vi "test-swerve-drve-odometry-01.vi"() -> (3 "Test Passed":bool)   [LabVIEW 2019]
uses:
  <vilib>/Rock Robotics/WPI/ThirdParty/JAS_Junk/TrajLib/TypeDef/SWERVE_DRIVE_ODOMETRY.ctl
  <vilib>/Rock Robotics/WPI/ThirdParty/JAS_Junk/TrajLib/TypeDef/POSE2D.ctl
  <vilib>/Rock Robotics/WPI/ThirdParty/JAS_Junk/TrajLib/TypeDef/TRANSLATION2D.ctl
  <vilib>/Rock Robotics/WPI/ThirdParty/JAS_Junk/TrajLib/TypeDef/ROTATION2D.ctl
  <vilib>/Rock Robotics/WPI/ThirdParty/JAS_Junk/TrajLib/TypeDef/SWERVE_DRIVE_MODULE_POSITION.ctl
  <vilib>/Rock Robotics/WPI/ThirdParty/JAS_Junk/TrajLib/TypeDef/SWERVE_DRIVE_KINEMATICS.ctl
  <vilib>/Analysis/Matrix/Datatypes/RealMatrix.ctl
  <vilib>/Rock Robotics/WPI/ThirdParty/JAS_Junk/TrajLib/TypeDef/SWERVE_DRIVE_MODULE_STATE.ctl
  <vilib>/Rock Robotics/WPI/ThirdParty/JAS_Junk/TrajLib/Conv_Deg_Radians.vi
  <vilib>/Rock Robotics/WPI/ThirdParty/JAS_Junk/TrajLib/Rotation2d_CreateAngle.vi
  <vilib>/Rock Robotics/WPI/ThirdParty/JAS_Junk/TrajLib/Trajectory_Library.lvlib
  <vilib>/Analysis/Matrix/NI_Matrix.lvlib
panel:
  out "Odom 1":T1={"POSE"={"TRANSLATION"={"X"=0.0, "Y"=0.0}, "ROTATION"={"VALUE"=0.0, "COS"=1.0, "SIN"=0.0}}, "GyroOffset"={"VALUE"=0.0, "COS"=1.0, "SIN"=0.0}, "PreviousAngle"={"VALUE"=0.0, "COS"=1.0, "SIN"=0.0}, "PrevModulePositions"=[], "NumModules"=0} {"PrevModulePositions"."Angle"."SIN" format="%13.4f"; "PrevModulePositions"."Angle"."COS" format="%13.4f"; "PrevModulePositions"."Angle"."VALUE" format="%13.4f"; "PreviousAngle"."SIN" format="%13.4f"; "PreviousAngle"."COS" format="%13.4f"; "PreviousAngle"."VALUE" format="%13.4f"; "GyroOffset"."SIN" format="%13.4f"; "GyroOffset"."COS" format="%13.4f"; "GyroOffset"."VALUE" format="%13.4f"; "POSE"."ROTATION"."SIN" format="%13.4f"; "POSE"."ROTATION"."COS" format="%13.4f"; "POSE"."ROTATION"."VALUE" format="%13.4f"; "POSE"."TRANSLATION"."Y" format="%14.3f"; "POSE"."TRANSLATION"."X" format="%14.3f"}
  out "robot POSE 4":T2={"TRANSLATION"={"X"=0.0, "Y"=0.0}, "ROTATION"={"VALUE"=0.0, "COS"=1.0, "SIN"=0.0}} {"ROTATION"."SIN" format="%13.4f"; "ROTATION"."COS" format="%13.4f"; "ROTATION"."VALUE" format="%13.4f"; "TRANSLATION"."Y" format="%14.3f"; "TRANSLATION"."X" format="%14.3f"}
  out "Odom 4":T1={"POSE"={"TRANSLATION"={"X"=0.0, "Y"=0.0}, "ROTATION"={"VALUE"=0.0, "COS"=1.0, "SIN"=0.0}}, "GyroOffset"={"VALUE"=0.0, "COS"=1.0, "SIN"=0.0}, "PreviousAngle"={"VALUE"=0.0, "COS"=1.0, "SIN"=0.0}, "PrevModulePositions"=[], "NumModules"=0} {"PrevModulePositions"."Angle"."SIN" format="%13.4f"; "PrevModulePositions"."Angle"."COS" format="%13.4f"; "PrevModulePositions"."Angle"."VALUE" format="%13.4f"; "PreviousAngle"."SIN" format="%13.4f"; "PreviousAngle"."COS" format="%13.4f"; "PreviousAngle"."VALUE" format="%13.4f"; "GyroOffset"."SIN" format="%13.4f"; "GyroOffset"."COS" format="%13.4f"; "GyroOffset"."VALUE" format="%13.4f"; "POSE"."ROTATION"."SIN" format="%13.4f"; "POSE"."ROTATION"."COS" format="%13.4f"; "POSE"."ROTATION"."VALUE" format="%13.4f"; "POSE"."TRANSLATION"."Y" format="%14.3f"; "POSE"."TRANSLATION"."X" format="%14.3f"}
  out "SWERVE_DRIVE_KINEMATICS":T6 {"SavedModuleStates"."Angle"."SIN" format="%13.4f"; "SavedModuleStates"."Angle"."COS" format="%13.4f"; "SavedModuleStates"."Angle"."VALUE" format="%13.4f"; "PrevCoR"."Y" format="%14.3f"; "PrevCoR"."X" format="%14.3f"; "Modules"."Y" format="%14.3f"; "Modules"."X" format="%14.3f"}
  out "robot POSE 3":T2={"TRANSLATION"={"X"=0.0, "Y"=0.0}, "ROTATION"={"VALUE"=0.0, "COS"=1.0, "SIN"=0.0}} {"ROTATION"."SIN" format="%13.4f"; "ROTATION"."COS" format="%13.4f"; "ROTATION"."VALUE" format="%13.4f"; "TRANSLATION"."Y" format="%14.3f"; "TRANSLATION"."X" format="%14.3f"}
  out "Odom 3":T1={"POSE"={"TRANSLATION"={"X"=0.0, "Y"=0.0}, "ROTATION"={"VALUE"=0.0, "COS"=1.0, "SIN"=0.0}}, "GyroOffset"={"VALUE"=0.0, "COS"=1.0, "SIN"=0.0}, "PreviousAngle"={"VALUE"=0.0, "COS"=1.0, "SIN"=0.0}, "PrevModulePositions"=[], "NumModules"=0} {"PrevModulePositions"."Angle"."SIN" format="%13.4f"; "PrevModulePositions"."Angle"."COS" format="%13.4f"; "PrevModulePositions"."Angle"."VALUE" format="%13.4f"; "PreviousAngle"."SIN" format="%13.4f"; "PreviousAngle"."COS" format="%13.4f"; "PreviousAngle"."VALUE" format="%13.4f"; "GyroOffset"."SIN" format="%13.4f"; "GyroOffset"."COS" format="%13.4f"; "GyroOffset"."VALUE" format="%13.4f"; "POSE"."ROTATION"."SIN" format="%13.4f"; "POSE"."ROTATION"."COS" format="%13.4f"; "POSE"."ROTATION"."VALUE" format="%13.4f"; "POSE"."TRANSLATION"."Y" format="%14.3f"; "POSE"."TRANSLATION"."X" format="%14.3f"}
  out "Odom 0":T1={"POSE"={"TRANSLATION"={"X"=0.0, "Y"=0.0}, "ROTATION"={"VALUE"=0.0, "COS"=1.0, "SIN"=0.0}}, "GyroOffset"={"VALUE"=0.0, "COS"=1.0, "SIN"=0.0}, "PreviousAngle"={"VALUE"=0.0, "COS"=1.0, "SIN"=0.0}, "PrevModulePositions"=[], "NumModules"=0} {"PrevModulePositions"."Angle"."SIN" format="%13.4f"; "PrevModulePositions"."Angle"."COS" format="%13.4f"; "PrevModulePositions"."Angle"."VALUE" format="%13.4f"; "PreviousAngle"."SIN" format="%13.4f"; "PreviousAngle"."COS" format="%13.4f"; "PreviousAngle"."VALUE" format="%13.4f"; "GyroOffset"."SIN" format="%13.4f"; "GyroOffset"."COS" format="%13.4f"; "GyroOffset"."VALUE" format="%13.4f"; "POSE"."ROTATION"."SIN" format="%13.4f"; "POSE"."ROTATION"."COS" format="%13.4f"; "POSE"."ROTATION"."VALUE" format="%13.4f"; "POSE"."TRANSLATION"."Y" format="%14.3f"; "POSE"."TRANSLATION"."X" format="%14.3f"}
  out "robot POSE 0":T2={"TRANSLATION"={"X"=0.0, "Y"=0.0}, "ROTATION"={"VALUE"=0.0, "COS"=1.0, "SIN"=0.0}} {"ROTATION"."SIN" format="%13.4f"; "ROTATION"."COS" format="%13.4f"; "ROTATION"."VALUE" format="%13.4f"; "TRANSLATION"."Y" format="%14.3f"; "TRANSLATION"."X" format="%14.3f"}
  out "robot POSE 1":T2={"TRANSLATION"={"X"=0.0, "Y"=0.0}, "ROTATION"={"VALUE"=0.0, "COS"=1.0, "SIN"=0.0}} {"ROTATION"."SIN" format="%13.4f"; "ROTATION"."COS" format="%13.4f"; "ROTATION"."VALUE" format="%13.4f"; "TRANSLATION"."Y" format="%14.3f"; "TRANSLATION"."X" format="%14.3f"}
  out "robot POSE 2":T2={"TRANSLATION"={"X"=0.0, "Y"=0.0}, "ROTATION"={"VALUE"=0.0, "COS"=1.0, "SIN"=0.0}} {"ROTATION"."SIN" format="%13.4f"; "ROTATION"."COS" format="%13.4f"; "ROTATION"."VALUE" format="%13.4f"; "TRANSLATION"."Y" format="%14.3f"; "TRANSLATION"."X" format="%14.3f"}
  out "Odom 2":T1={"POSE"={"TRANSLATION"={"X"=0.0, "Y"=0.0}, "ROTATION"={"VALUE"=0.0, "COS"=1.0, "SIN"=0.0}}, "GyroOffset"={"VALUE"=0.0, "COS"=1.0, "SIN"=0.0}, "PreviousAngle"={"VALUE"=0.0, "COS"=1.0, "SIN"=0.0}, "PrevModulePositions"=[], "NumModules"=0} {"PrevModulePositions"."Angle"."SIN" format="%13.4f"; "PrevModulePositions"."Angle"."COS" format="%13.4f"; "PrevModulePositions"."Angle"."VALUE" format="%13.4f"; "PreviousAngle"."SIN" format="%13.4f"; "PreviousAngle"."COS" format="%13.4f"; "PreviousAngle"."VALUE" format="%13.4f"; "GyroOffset"."SIN" format="%13.4f"; "GyroOffset"."COS" format="%13.4f"; "GyroOffset"."VALUE" format="%13.4f"; "POSE"."ROTATION"."SIN" format="%13.4f"; "POSE"."ROTATION"."COS" format="%13.4f"; "POSE"."ROTATION"."VALUE" format="%13.4f"; "POSE"."TRANSLATION"."Y" format="%14.3f"; "POSE"."TRANSLATION"."X" format="%14.3f"}
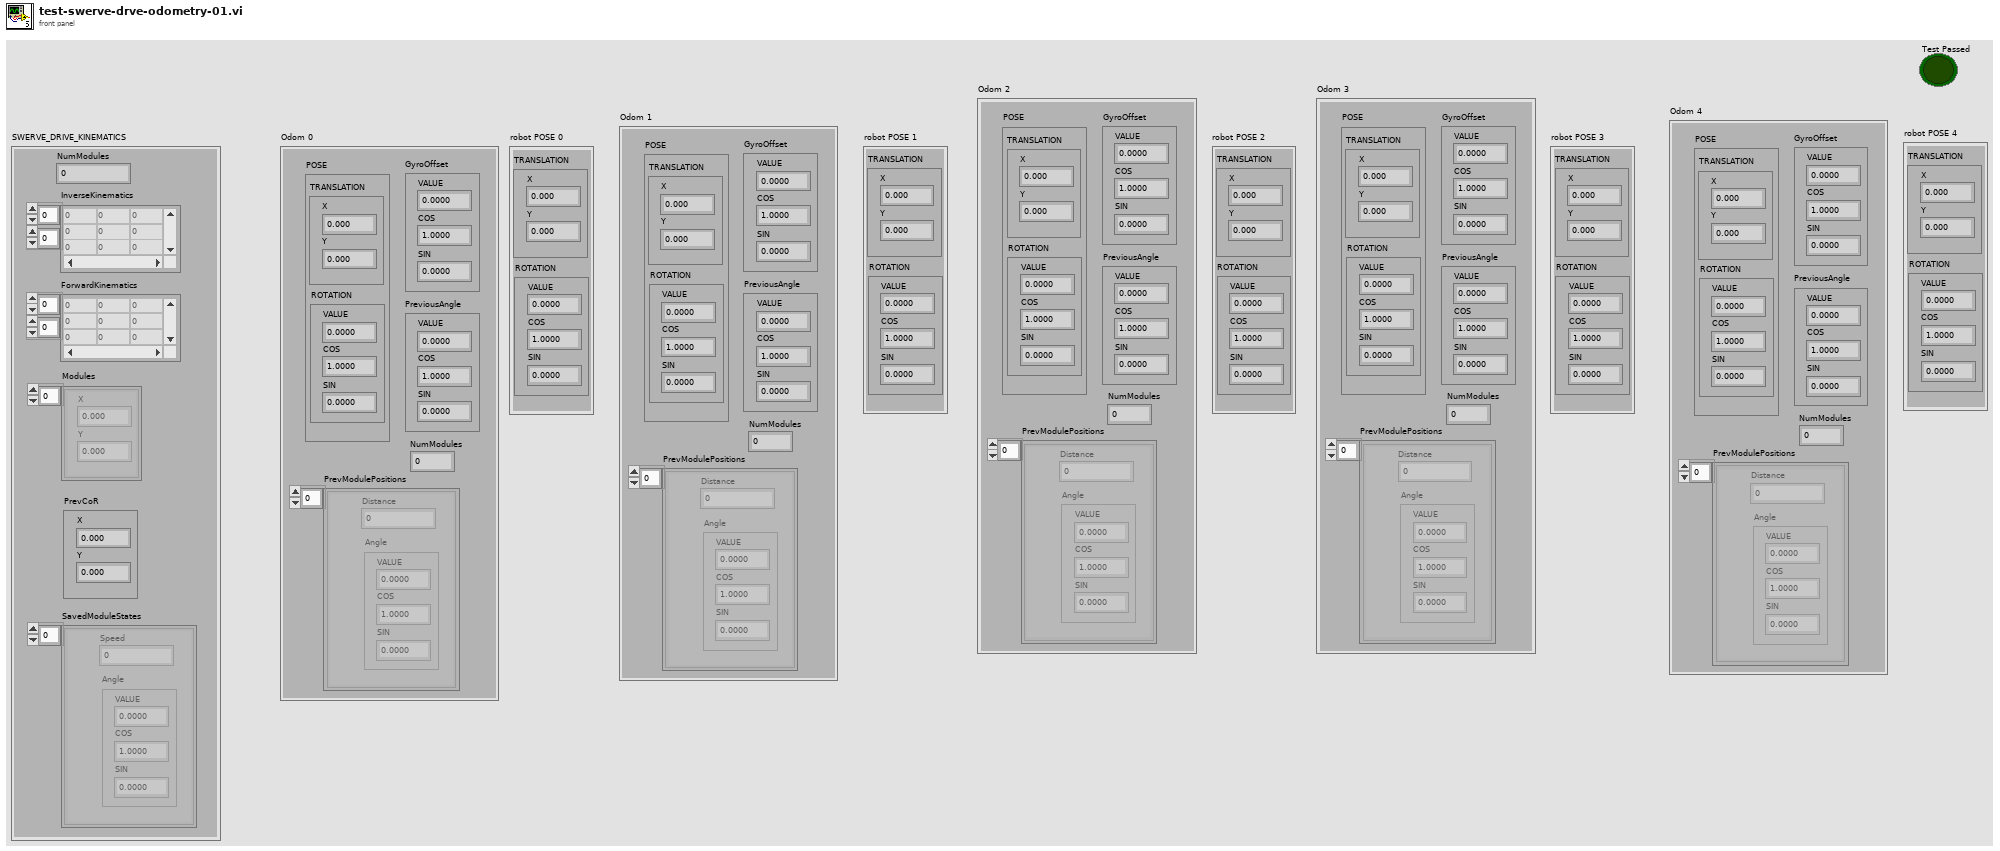
[diagram p1: front panel]
types:
  T1 = typedef "Trajectory_Library.lvlib/SWERVE_DRIVE_ODOMETRY.ctl" = cluster{"POSE":T2, "GyroOffset":T4, "PreviousAngle":T4, "PrevModulePositions":T5[], "NumModules":i32}
  T2 = typedef "Trajectory_Library.lvlib/POSE2D.ctl" = cluster{"TRANSLATION":T3, "ROTATION":T4}
  T3 = typedef "Trajectory_Library.lvlib/TRANSLATION2D.ctl" = cluster{"X":dbl, "Y":dbl}
  T4 = typedef "Trajectory_Library.lvlib/ROTATION2D.ctl" = cluster{"VALUE":dbl, "COS":dbl, "SIN":dbl}
  T5 = typedef "Trajectory_Library.lvlib/SWERVE_DRIVE_MODULE_POSITION.ctl" = cluster{"Distance":dbl, "Angle":T4}
  T6 = typedef "Trajectory_Library.lvlib/SWERVE_DRIVE_KINEMATICS.ctl" = cluster{"NumModules":i32, "InverseKinematics":T7, "ForwardKinematics":T7, "Modules":T3[], "PrevCoR":T3, "SavedModuleStates":T8[]}
  T7 = typedef "NI_Matrix.lvlib/RealMatrix.ctl" = dbl[][]
  T8 = typedef "Trajectory_Library.lvlib/SWERVE_DRIVE_MODULE_STATE.ctl" = cluster{"Speed":dbl, "Angle":T4}
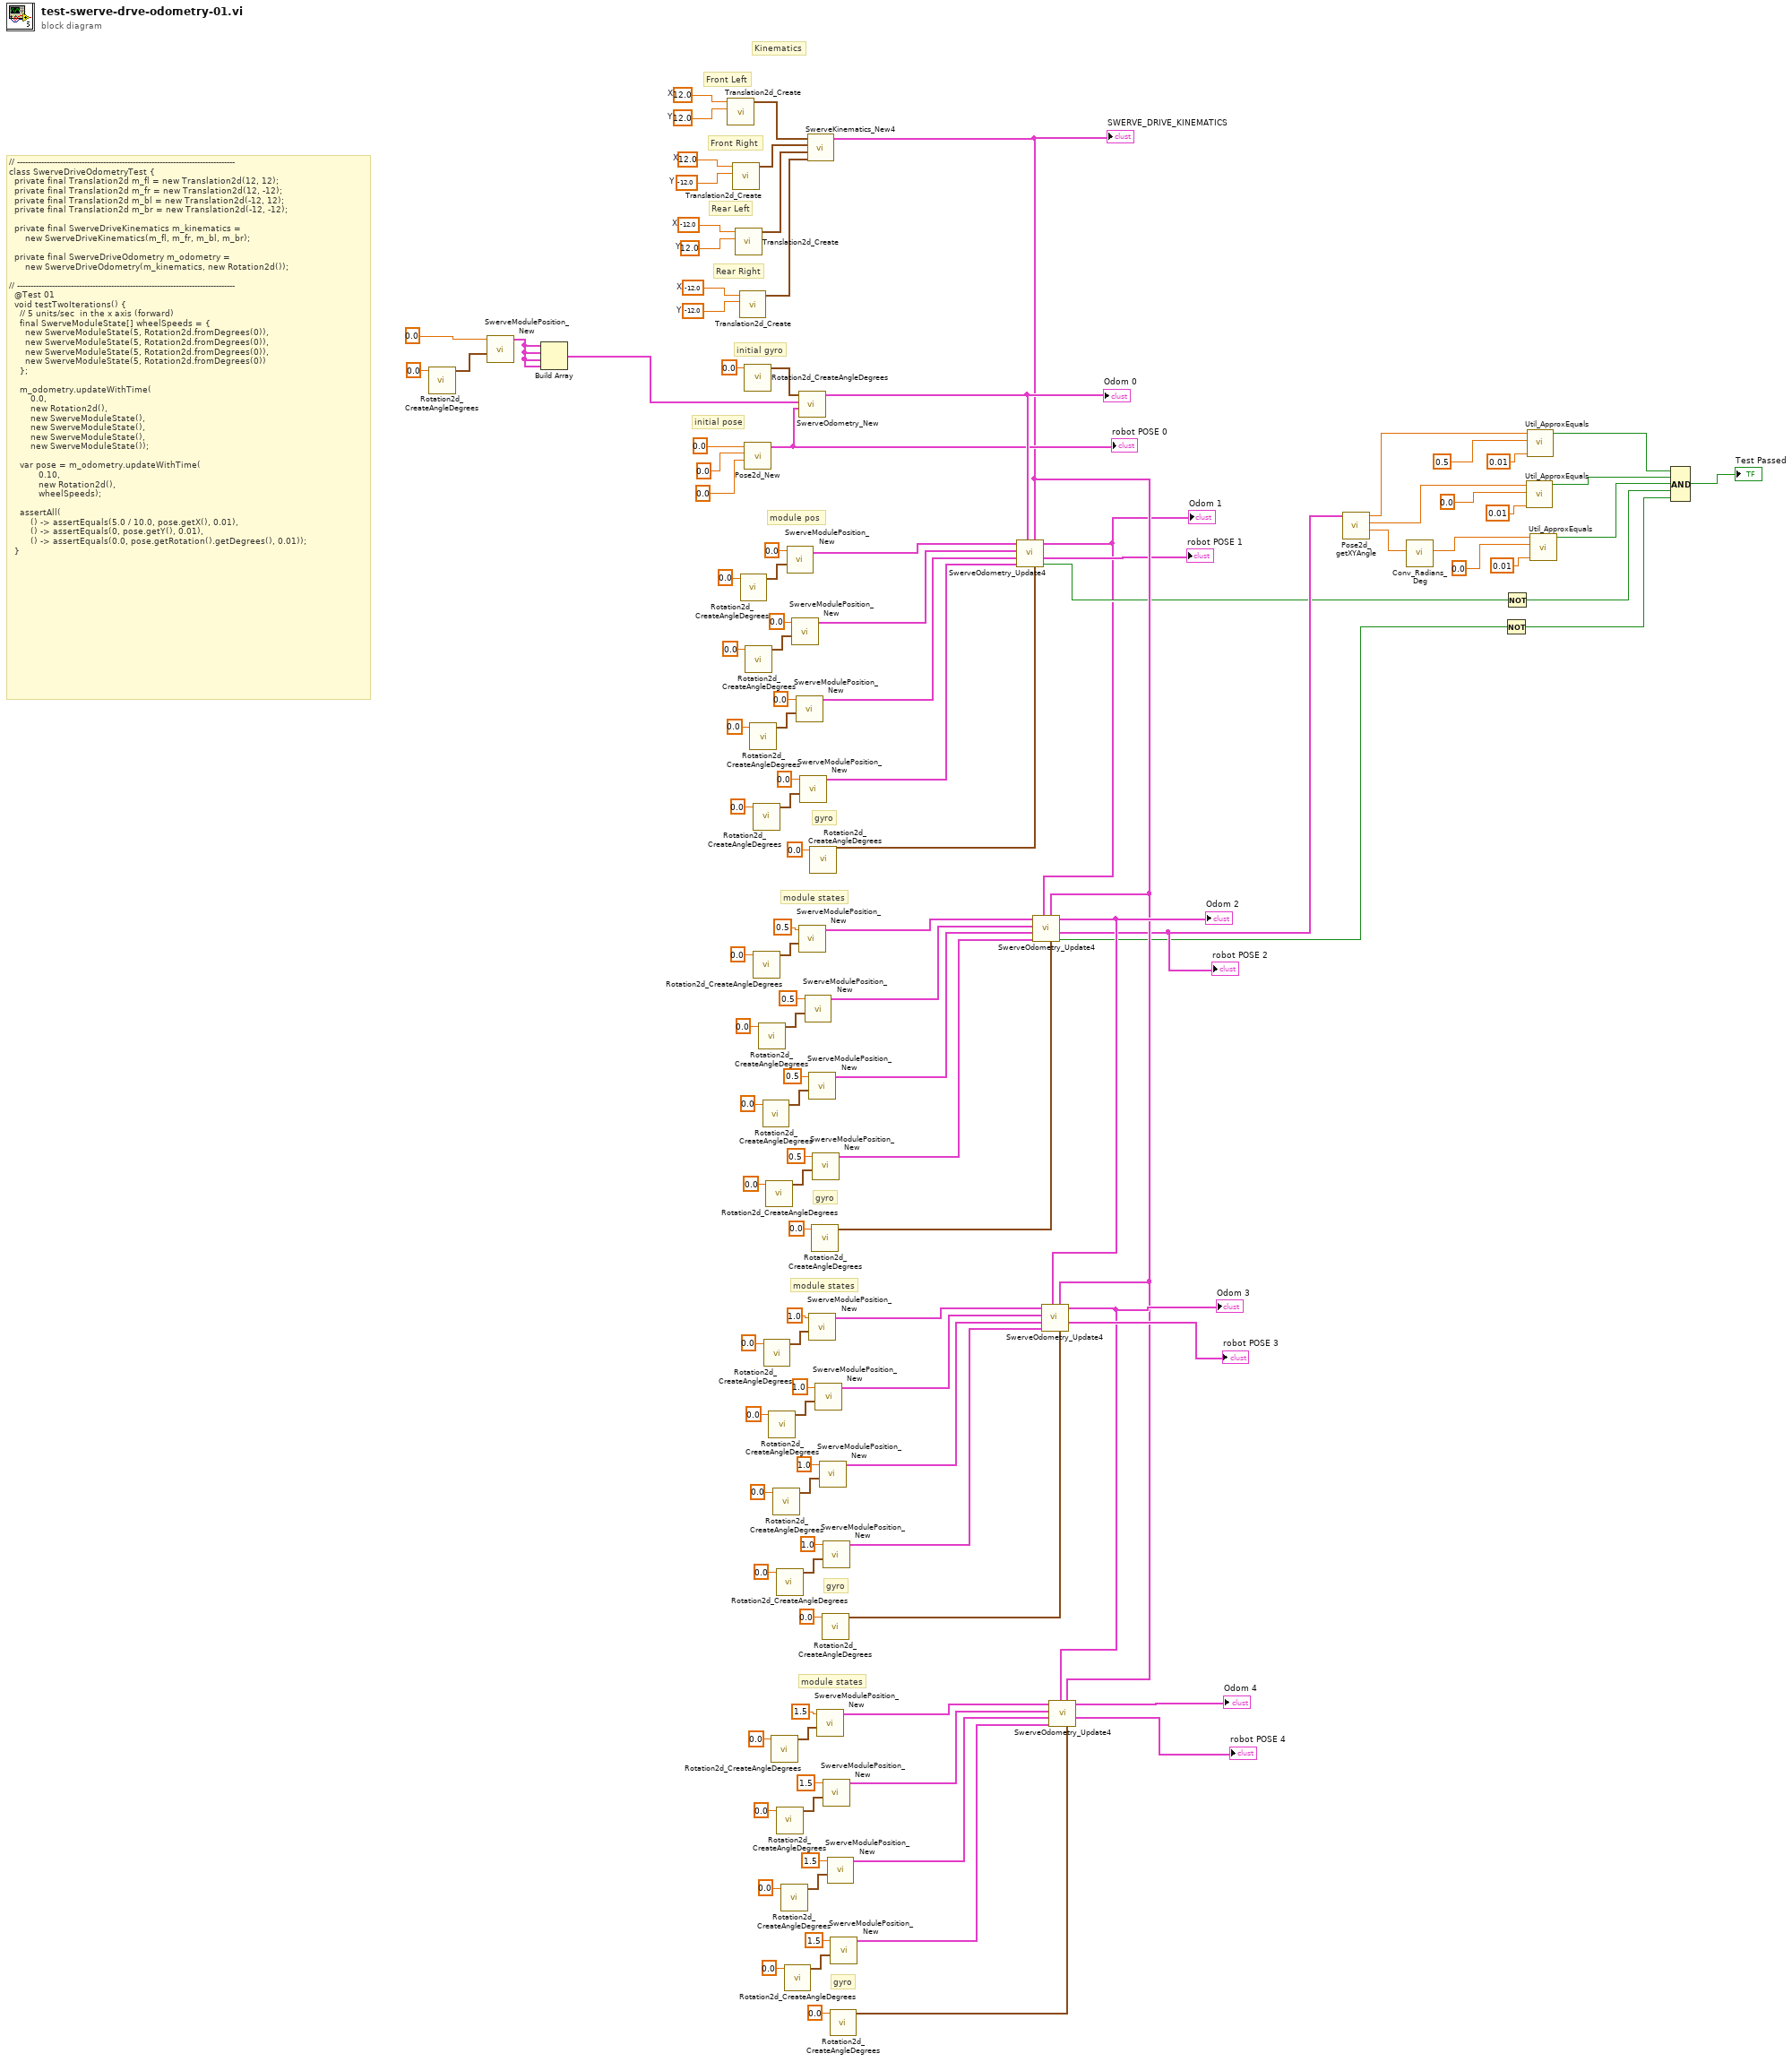
[diagram p0: block diagram]
diagram:
  w119 = -12.0  # X
  w118 = -12.0  # Y
  w117 = -12.0  # X
  w116 = 12.0  # Y
  w115 = 12.0  # X
  w114 = -12.0  # Y
  w113 = 12.0  # X
  w112 = 12.0  # Y
  # "gyro"
  # "module states"
  # "gyro"
  # "module states"
  # "initial pose"
  # "gyro"
  # "module states"
  # "gyro"
  # "module pos"
  # "Kinematics"
  # "initial gyro"
  # "Rear Right"
  # "Rear Left"
  # "Front Right"
  # "Front Left"
  # "// ---------------------------------------------------------------------------------\nclass SwerveDriveOdometryTest {\n  private final Translation2d m_fl = new Translation2d(12, 12);\n  private final Translation2d m_fr = new Translation2d(12, -12);\n  private final Translation2d m_bl = new Translation2d(-12, 12);\n  private final Translation2d m_br = new Translation2d(-12, -12);\n\n  private final SwerveDriveKinematics m_kinematics =\n      new SwerveDriveKinematics(m_fl, m_fr, m_bl, m_br);\n\n  private final SwerveDriveOdometry m_odometry =\n      new SwerveDriveOdometry(m_kinematics, new Rotation2d());\n\n// ---------------------------------------------------------------------------------\n  @Test 01\n  void testTwoIterations() {\n    // 5 units/sec  in the x axis (forward)\n    final SwerveModuleState[] wheelSpeeds = {\n      new SwerveModuleState(5, Rotation2d.fromDegrees(0)),\n      new SwerveModuleState(5, Rotation2d.fromDegrees(0)),\n      new SwerveModuleState(5, Rotation2d.fromDegrees(0)),\n      new SwerveModuleState(5, Rotation2d.fromDegrees(0))\n    };\n\n    m_odometry.updateWithTime(\n        0.0,\n        new Rotation2d(),\n        new SwerveModuleState(),\n        new SwerveModuleState(),\n        new SwerveModuleState(),\n        new SwerveModuleState());\n\n    var pose = m_odometry.updateWithTime(\n           0.10, \n           new Rotation2d(), \n           wheelSpeeds);\n\n    assertAll(\n        () -> assertEquals(5.0 / 10.0, pose.getX(), 0.01),\n        () -> assertEquals(0, pose.getY(), 0.01),\n        () -> assertEquals(0.0, pose.getRotation().getDegrees(), 0.01));\n  }"
  n1 = call <vilib>:"Rotation2d_CreateAngleDegrees.vi"("Angle_Degrees"=0.0) -> ("ROTATION"=w9:T4)  [unwired: 10 in]
  n2 = call <vilib>:"SwerveModulePosition_New.vi"("ROTATION"=w9, "Distance"=0.0) -> ("SWERVE_DRIVE_MODULE_POSITION"=w7:T5)  [unwired: 9 in]
  n3 = Build Array(w7, w7, w7, w7) -> (w6:T5[])
  n4 = call <vilib>:"Translation2d_Create.vi"("Y"=w112, "X"=w113) -> ("TRANSLATION"=w120:T3)  [unwired: 9 in]
  n5 = call <vilib>:"Translation2d_Create.vi"("Y"=w114, "X"=w115) -> ("TRANSLATION"=w121:T3)  [unwired: 9 in]
  n6 = call <vilib>:"Translation2d_Create.vi"("Y"=w116, "X"=w117) -> ("TRANSLATION"=w122:T3)  [unwired: 9 in]
  n7 = call <vilib>:"Translation2d_Create.vi"("Y"=w118, "X"=w119) -> ("TRANSLATION"=w123:T3)  [unwired: 9 in]
  n8 = call <vilib>:"Rotation2d_CreateAngleDegrees.vi"("Angle_Degrees"=0.0) -> ("ROTATION"=w105:T4)  [unwired: 10 in]
  n9 = call <vilib>:"Rotation2d_CreateAngleDegrees.vi"("Angle_Degrees"=0.0) -> ("ROTATION"=w108:T4)  [unwired: 10 in]
  n10 = call <vilib>:"Pose2d_New.vi"("Heading"=0.0, "Y"=0.0, "X"=0.0) -> ("out POSe"=w69:T2)  [unwired: 8 in]
  "robot POSE 0" <- w69
  n11 = call <vilib>:"Rotation2d_CreateAngleDegrees.vi"("Angle_Degrees"=0.0) -> ("ROTATION"=w102:T4)  [unwired: 10 in]
  n12 = call <vilib>:"Rotation2d_CreateAngleDegrees.vi"("Angle_Degrees"=0.0) -> ("ROTATION"=w99:T4)  [unwired: 10 in]
  n13 = call <vilib>:"Rotation2d_CreateAngleDegrees.vi"("Angle_Degrees"=0.0) -> ("ROTATION"=w96:T4)  [unwired: 10 in]
  n14 = call <vilib>:"Rotation2d_CreateAngleDegrees.vi"("Angle_Degrees"=0.0) -> ("ROTATION"=w89:T4)  [unwired: 10 in]
  n15 = call <vilib>:"Rotation2d_CreateAngleDegrees.vi"("Angle_Degrees"=0.0) -> ("ROTATION"=w86:T4)  [unwired: 10 in]
  n16 = call <vilib>:"Rotation2d_CreateAngleDegrees.vi"("Angle_Degrees"=0.0) -> ("ROTATION"=w83:T4)  [unwired: 10 in]
  n17 = call <vilib>:"Rotation2d_CreateAngleDegrees.vi"("Angle_Degrees"=0.0) -> ("ROTATION"=w67:T4)  [unwired: 10 in]
  n18 = call <vilib>:"Rotation2d_CreateAngleDegrees.vi"("Angle_Degrees"=0.0) -> ("ROTATION"=w80:T4)  [unwired: 10 in]
  n19 = call <vilib>:"Rotation2d_CreateAngleDegrees.vi"("Angle_Degrees"=0.0) -> ("ROTATION"=w64:T4)  [unwired: 10 in]
  n20 = call <vilib>:"Rotation2d_CreateAngleDegrees.vi"("Angle_Degrees"=0.0) -> ("ROTATION"=w47:T4)  [unwired: 10 in]
  n21 = call <vilib>:"Rotation2d_CreateAngleDegrees.vi"("Angle_Degrees"=0.0) -> ("ROTATION"=w61:T4)  [unwired: 10 in]
  n22 = call <vilib>:"Rotation2d_CreateAngleDegrees.vi"("Angle_Degrees"=0.0) -> ("ROTATION"=w58:T4)  [unwired: 10 in]
  n23 = call <vilib>:"Rotation2d_CreateAngleDegrees.vi"("Angle_Degrees"=0.0) -> ("ROTATION"=w44:T4)  [unwired: 10 in]
  n24 = call <vilib>:"Rotation2d_CreateAngleDegrees.vi"("Angle_Degrees"=0.0) -> ("ROTATION"=w41:T4)  [unwired: 10 in]
  n25 = call <vilib>:"Rotation2d_CreateAngleDegrees.vi"("Angle_Degrees"=0.0) -> ("ROTATION"=w38:T4)  [unwired: 10 in]
  n26 = call <vilib>:"SwerveModulePosition_New.vi"("ROTATION"=w105, "Distance"=0.0 ("Speed")) -> ("SWERVE_DRIVE_MODULE_POSITION"=w94:T5)  [unwired: 9 in]
  n27 = call <vilib>:"SwerveModulePosition_New.vi"("ROTATION"=w102, "Distance"=0.0 ("Speed")) -> ("SWERVE_DRIVE_MODULE_POSITION"=w93:T5)  [unwired: 9 in]
  n28 = call <vilib>:"SwerveModulePosition_New.vi"("ROTATION"=w99, "Distance"=0.0 ("Speed")) -> ("SWERVE_DRIVE_MODULE_POSITION"=w92:T5)  [unwired: 9 in]
  n29 = call <vilib>:"SwerveOdometry_New.vi"("InitialPose"=w69, "Module Positions"=w6, "gyroAngle"=w108) -> ("SWERVE_DRIVE_ODOMETRY"=w70:T1)  [unwired: 8 in]
  "Odom 0" <- w70
  n30 = call <vilib>:"SwerveModulePosition_New.vi"("ROTATION"=w89, "Distance"=0.5 ("Speed")) -> ("SWERVE_DRIVE_MODULE_POSITION"=w78:T5)  [unwired: 9 in]
  n31 = call <vilib>:"SwerveModulePosition_New.vi"("ROTATION"=w96, "Distance"=0.0 ("Speed")) -> ("SWERVE_DRIVE_MODULE_POSITION"=w91:T5)  [unwired: 9 in]
  n32 = call <vilib>:"SwerveModulePosition_New.vi"("ROTATION"=w86, "Distance"=0.5 ("Speed")) -> ("SWERVE_DRIVE_MODULE_POSITION"=w77:T5)  [unwired: 9 in]
  n33 = call <vilib>:"SwerveKinematics_New4.vi"("wheel 3"=w123, "wheel 2"=w122, "wheel 1"=w121, "wheel 0"=w120) -> ("SWERVE_DRIVE_KINEMATICS"=w27:T6)  [unwired: 7 in]
  "SWERVE_DRIVE_KINEMATICS" <- w27
  n34 = call <vilib>:"SwerveModulePosition_New.vi"("ROTATION"=w83, "Distance"=0.5 ("Speed")) -> ("SWERVE_DRIVE_MODULE_POSITION"=w76:T5)  [unwired: 9 in]
  n35 = call <vilib>:"SwerveModulePosition_New.vi"("ROTATION"=w67, "Distance"=1.0 ("Speed")) -> ("SWERVE_DRIVE_MODULE_POSITION"=w56:T5)  [unwired: 9 in]
  n36 = call <vilib>:"Rotation2d_CreateAngleDegrees.vi"("Angle_Degrees"=0.0) -> ("ROTATION"=w73:T4)  [unwired: 10 in]
  n37 = call <vilib>:"Rotation2d_CreateAngleDegrees.vi"("Angle_Degrees"=0.0) -> ("ROTATION"=w71:T4)  [unwired: 10 in]
  n38 = call <vilib>:"SwerveModulePosition_New.vi"("ROTATION"=w80, "Distance"=0.5 ("Speed")) -> ("SWERVE_DRIVE_MODULE_POSITION"=w75:T5)  [unwired: 9 in]
  n39 = call <vilib>:"SwerveModulePosition_New.vi"("ROTATION"=w64, "Distance"=1.0 ("Speed")) -> ("SWERVE_DRIVE_MODULE_POSITION"=w55:T5)  [unwired: 9 in]
  n40 = call <vilib>:"SwerveModulePosition_New.vi"("ROTATION"=w47, "Distance"=1.5 ("Speed")) -> ("SWERVE_DRIVE_MODULE_POSITION"=w36:T5)  [unwired: 9 in]
  n41 = call <vilib>:"SwerveModulePosition_New.vi"("ROTATION"=w61, "Distance"=1.0 ("Speed")) -> ("SWERVE_DRIVE_MODULE_POSITION"=w54:T5)  [unwired: 9 in]
  n42 = call <vilib>:"Rotation2d_CreateAngleDegrees.vi"("Angle_Degrees"=0.0) -> ("ROTATION"=w51:T4)  [unwired: 10 in]
  n43 = call <vilib>:"SwerveModulePosition_New.vi"("ROTATION"=w58, "Distance"=1.0 ("Speed")) -> ("SWERVE_DRIVE_MODULE_POSITION"=w53:T5)  [unwired: 9 in]
  n44 = call <vilib>:"SwerveModulePosition_New.vi"("ROTATION"=w44, "Distance"=1.5 ("Speed")) -> ("SWERVE_DRIVE_MODULE_POSITION"=w35:T5)  [unwired: 9 in]
  n45 = call <vilib>:"SwerveModulePosition_New.vi"("ROTATION"=w41, "Distance"=1.5 ("Speed")) -> ("SWERVE_DRIVE_MODULE_POSITION"=w34:T5)  [unwired: 9 in]
  n46 = call <vilib>:"Rotation2d_CreateAngleDegrees.vi"("Angle_Degrees"=0.0) -> ("ROTATION"=w31:T4)  [unwired: 10 in]
  n47 = call <vilib>:"SwerveModulePosition_New.vi"("ROTATION"=w38, "Distance"=1.5 ("Speed")) -> ("SWERVE_DRIVE_MODULE_POSITION"=w33:T5)  [unwired: 9 in]
  n48 = call <vilib>:"SwerveOdometry_Update4.vi"("gyroAngle"=w73, "SWERVE_DRIVE_KINEMATICS"=w27, "in SWERVE_DRIVE_ODOMETRY"=w70, "Wheel Position 3"=w91, "Wheel Position 2"=w92, "Wheel Position 1"=w93, "Wheel Position 0"=w94) -> ("Error"=w5:bool, "robot POSE"=→"robot POSE 1":T2, "out SWERVE_DRIVE_ODOMETRY"=w1:T1)  [unwired: 2 in]
  "Odom 1" <- w1
  n49 = call <vilib>:"SwerveOdometry_Update4.vi"("gyroAngle"=w71, "SWERVE_DRIVE_KINEMATICS"=w27, "in SWERVE_DRIVE_ODOMETRY"=w1, "Wheel Position 3"=w75, "Wheel Position 2"=w76, "Wheel Position 1"=w77, "Wheel Position 0"=w78) -> ("Error"=w2:bool, "robot POSE"=w11:T2, "out SWERVE_DRIVE_ODOMETRY"=w49:T1)  [unwired: 2 in]
  "Odom 2" <- w49
  "robot POSE 2" <- w11
  n50 = call <vilib>:"SwerveOdometry_Update4.vi"("gyroAngle"=w51, "SWERVE_DRIVE_KINEMATICS"=w27, "in SWERVE_DRIVE_ODOMETRY"=w49, "Wheel Position 3"=w53, "Wheel Position 2"=w54, "Wheel Position 1"=w55, "Wheel Position 0"=w56) -> ("robot POSE"=→"robot POSE 3":T2, "out SWERVE_DRIVE_ODOMETRY"=w28:T1)  [unwired: 2 in, 1 out]
  "Odom 3" <- w28
  n51 = call <vilib>:"SwerveOdometry_Update4.vi"("gyroAngle"=w31, "SWERVE_DRIVE_KINEMATICS"=w27, "in SWERVE_DRIVE_ODOMETRY"=w28, "Wheel Position 3"=w33, "Wheel Position 2"=w34, "Wheel Position 1"=w35, "Wheel Position 0"=w36) -> ("robot POSE"=→"robot POSE 4":T2, "out SWERVE_DRIVE_ODOMETRY"=→"Odom 4":T1)  [unwired: 2 in, 1 out]
  n52 = call <vilib>:"Pose2d_getXYAngle.vi"("in POSE"=w11) -> ("Angle"=w23:dbl, "Y"=w20:dbl, "X"=w21:dbl)  [unwired: 8 in]
  n53 = call <vilib>:"Conv_Radians_Deg.vi"("Radians"=w23) -> ("Degrees"=w19:dbl)  [unwired: 10 in]
  n54 = Not(x=w2) -> (.not. x?=w3:bool)
  n55 = Not(x=w5) -> (.not. x?=w4:bool)
  n56 = call <vilib>:"Util_ApproxEquals.vi"("Tolerance"=0.01, "Value 2"=0.0, "Value 1"=w20) -> ("ApproxEquals"=w14:bool)  [unwired: 8 in]
  n57 = call <vilib>:"Util_ApproxEquals.vi"("Tolerance"=0.01, "Value 2"=0.5, "Value 1"=w21) -> ("ApproxEquals"=w15:bool)  [unwired: 8 in]
  n58 = call <vilib>:"Util_ApproxEquals.vi"("Tolerance"=0.01, "Value 2"=0.0, "Value 1"=w19) -> ("ApproxEquals"=w13:bool)  [unwired: 8 in]
  n59 = Compound Arithmetic op=AND(w15, w14, w13, w4, w3) -> (→"Test Passed":bool)
